vi "Check Moving.vi"(8 "error in (no error)":errorcluster, 11 "FINE SIM Motion Axis":refnum<class "FINE SIM Motion Axis.lvclass">) -> (0 "error out":errorcluster, 3 "FINE SIM Motion Axis":refnum<class "FINE SIM Motion Axis.lvclass">)   [LabVIEW 2022 SP3, in "FINE SIM Motion Axis.lvclass"]
uses:
  FINE SIM Motion Axis.lvclass
  FINE SIM Motion Axis.lvclass/FINE SIM Motion Axis.ctl
  Accessors/Read Sim Axis Data.vi
  Accessors/Write Sim Axis Data.vi
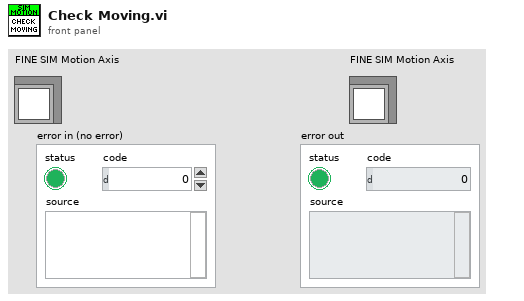
[diagram p1: front panel]
types:
  T1 = typedef "FINE SIM Motion Axis.lvclass/Axis Data.ctl" = cluster{"Axis Parameters":T2, "Axis Settings":T4, "Time Stamp":timestamp}
  T2 = typedef "FINE SIM Motion Axis.lvclass/Axis Parameters.ctl" = cluster{"Moving":bool, "Homed":bool, "Desired Position":dbl, "Current Positon":dbl, "Current Speed":dbl, "Home Status":T3}
  T3 = typedef "FINE SIM Motion Axis.lvclass/Homing Status.ctl" = enum16{"Idle", "Inital Home Motion", "Final Home Motion", "Done Homing"}
  T4 = typedef "FINE SIM Motion Axis.lvclass/Axis Settings.ctl" = cluster{"Speed":dbl, "Acceleration":dbl}
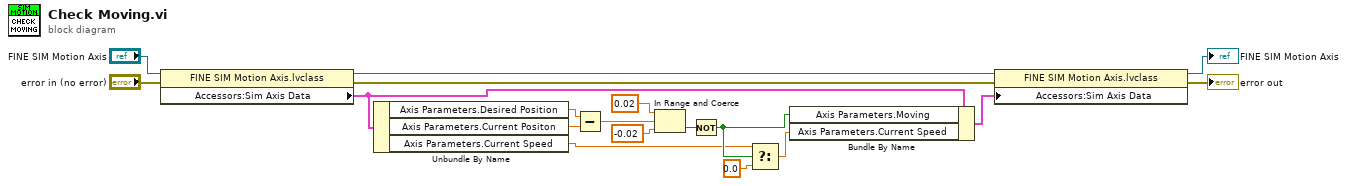
[diagram p0: block diagram]
diagram:
  n1 = property class="FINE SIM Motion Axis.lvclass"(reference="FINE SIM Motion Axis", error in="error in (no error)") -> (reference out=w9:refnum<class "FINE SIM Motion Axis.lvclass">, error out=w17:errorcluster, "Accessors:Sim Axis Data"=w7:T1)
  n2 = Unbundle By Name(w7) -> ("Axis Parameters.Desired Position"=w11:dbl, "Axis Parameters.Current Positon"=w12:dbl, "Axis Parameters.Current Speed"=w5:dbl)
  n3 = Subtract(x=w11, y=w12) -> (x-y=w13:dbl)
  n4 = In Range and Coerce(upper limit=0.02, x=w13, lower limit=-0.02) -> (In Range?=w16:bool)  [unwired: 1 out]
  n5 = Not(x=w16) -> (.not. x?=w6:bool)
  n6 = Select(t=w5, s=w6, f=0.0) -> (s? t:f=w4:dbl)
  n7 = Bundle By Name(cluster=w7, "Axis Parameters.Moving"=w6, "Axis Parameters.Current Speed"=w4) -> (w8:T1)
  n8 = property class="FINE SIM Motion Axis.lvclass"(reference=w9, error in=w17, "Accessors:Sim Axis Data"=w8) -> (reference out=→"FINE SIM Motion Axis":refnum<class "FINE SIM Motion Axis.lvclass">, error out=→"error out":errorcluster)
